vi "Read VI Store.vi"(8 "error in (no error)":errorcluster, 11 "Settings in":refnum<class "Settings.lvclass">) -> (0 "error out":errorcluster, 2 "VI App Store.lvlib:VIStore.lvclass":refnum<class "VIStore.lvclass">, 3 "Settings out":refnum<class "Settings.lvclass">)   [LabVIEW 2015, in "Item Actor.lvlib" / "Settings.lvclass"]
uses:
  Settings.lvclass
  VI Store/VIStore Actor/VIStore.lvclass
  Settings.lvclass/Settings.ctl
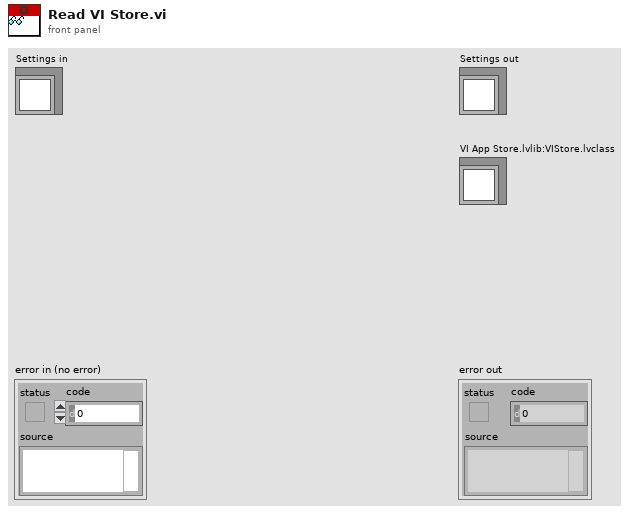
[diagram p1: front panel]
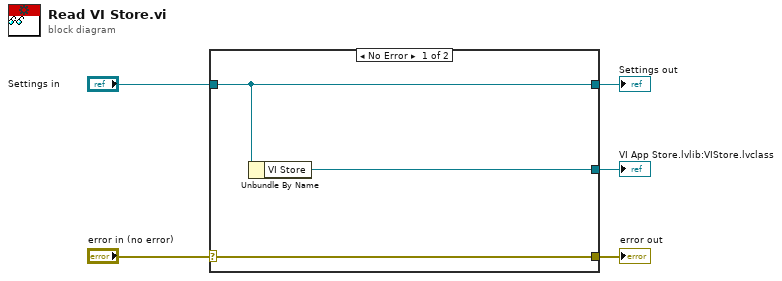
[diagram p0: block diagram]
diagram:
  n1 = case shown="No Error" "error in (no error)" {
    selector: "error in (no error)" -> [w8 w9]
    tunnel: [w8 w9] -> w4
    tunnel: [w7 w10] -> w2
    tunnel: "Settings in" -> [w7 w10]
    tunnel: [w6 _] -> w1
    frame No Error {
      n2 = Unbundle By Name(w7) -> ("VI Store"=w6:refnum<class "VIStore.lvclass">)
    }
    frame Error {
    }
  }
  "error out" <- w4
  "Settings out" <- w2
  "VI App Store.lvlib:VIStore.lvclass" <- w1
